vi "svmdense_predict_values.vi"(8 "error in (no error)":errorcluster, 10 "x":dbl[](array[numeric]), 11 "Model":T1) -> (0 "error out":errorcluster, 2 "Decision values":dbl[](array[numeric]), 3 "Predicted label":dbl)   [LabVIEW 2015]
doc: "This function gives decision values on a test vector x given a model, and return the predicted label (classification) or the function value (regression).\n\nFor a classification model with nr_class classes, this function gives nr_class*(nr_class-1)/2 decision values in the output array. The order is \nlabel[0] vs. label[1], ..., label[0] vs. label[nr_class-1], \nlabel[1] vs. label[2], ..., label[nr_class-2] vs. label[nr_class-1], \nThe labels are contained within the model. The returned value is the predicted class for x. Note that when nr_class = 1, this function does not give any decision value.\n\nFor a regression model, dec_values[0] and the returned value are both the function value of x calculated using the model. For a one-class model, dec_values[0] is the decision value of x, while the returned value is +1/-1."
uses:
  Controls/svmdense_model.ctl
  LibSVM Sparse/Wrapper API/Controls/svm_parameter.ctl
  LibSVM Sparse/Wrapper API/Controls/svm_type.ctl
  LibSVM Sparse/Wrapper API/Controls/svm_kernel_type.ctl
  bin/x64/LabVIEW-libsvm-dense.dll
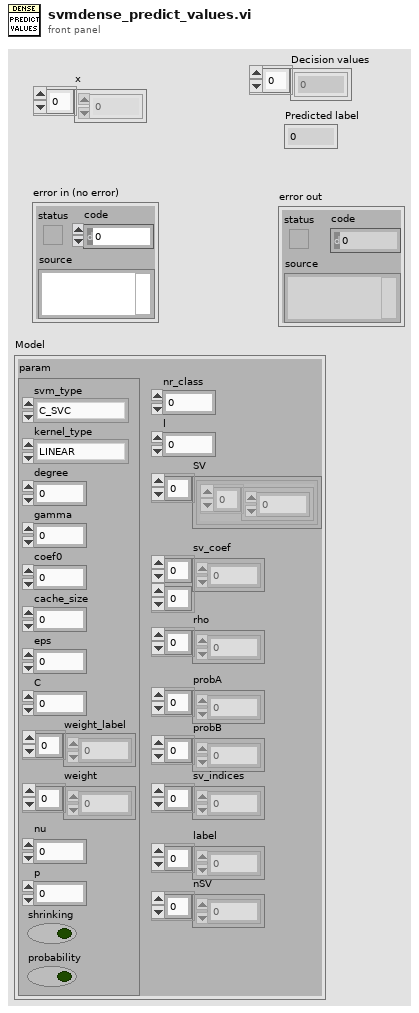
[diagram p1: front panel]
types:
  T1 = typedef "svmdense_model.ctl" = cluster{"param":T2, "nr_class":i32, "l":i32, "SV":cluster{"Array":dbl[]}[], "sv_coef":dbl[][], "rho":dbl[], "probA":dbl[], "probB":dbl[], "sv_indices":i32[], "label":i32[], "nSV":i32[]}
  T2 = typedef "svm_parameter.ctl" = cluster{"svm_type":T3, "kernel_type":T4, "degree":i32, "gamma":dbl, "coef0":dbl, "cache_size":dbl, "eps":dbl, "C":dbl, "weight_label":i32[], "weight":dbl[], "nu":dbl, "p":dbl, "shrinking":bool, "probability":bool}
  T3 = typedef "svm_type.ctl" = enum32{"C_SVC", "NU_SVC", "ONE_CLASS", "EPSILON_SVR", "NU_SVR"}
  T4 = typedef "svm_kernel_type.ctl" = enum32{"LINEAR", "POLY", "RBF", "SIGMOID", "PRECOMPUTED"}
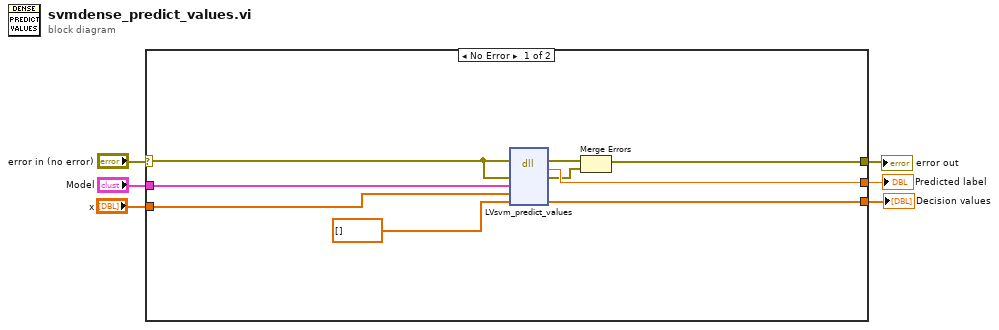
[diagram p0: block diagram]
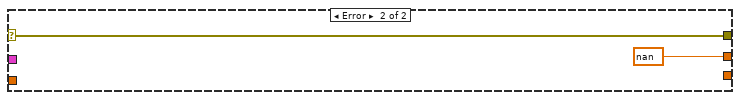
[diagram p2: hidden frame]
diagram:
  n1 = case shown="No Error" "error in (no error)" {
    selector: "error in (no error)" -> [w15 w17]
    tunnel: [w14 w17] -> w6
    tunnel: "Model" -> [w13 _]
    tunnel: "x" -> [w12 _]
    tunnel: [w11 nan ("predicted label")] -> w4
    tunnel: [w10 _] -> w3
    frame No Error {
      n2 = dll-call lib="C:/dev/LabVIEW-libsvm/LabVIEW/bin/x64/LabVIEW-libsvm-dense.*" fn="LVsvm_predict_values"(error in=w15, "lvErr"=w15, "model_in"=w13, "x_in"=w12, "dec_values_out"=dbl[] []) -> (error out=w9:errorcluster, "predicted label"=w11:dbl, "lvErr"=w8:errorcluster, "dec_values_out"=w10:dbl[])  [unwired: 4 in, 1 out]
      n3 = Merge Errors(w9, w8) -> (w14:errorcluster)
    }
    frame Error {
    }
  }
  "error out" <- w6
  "Predicted label" <- w4
  "Decision values" <- w3
